vi "Com_SECS Equipment _Session Read.vi"(8 "error in":errorcluster, 10 "Timeout(100)":i32=100, 11 "Session In":refnum<k5>) -> (0 "error out":errorcluster, 2 "Read Data":string, 3 "Session Out":refnum<k5>)   [LabVIEW 2016]
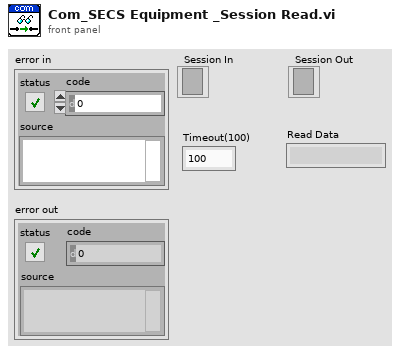
[diagram p1: front panel]
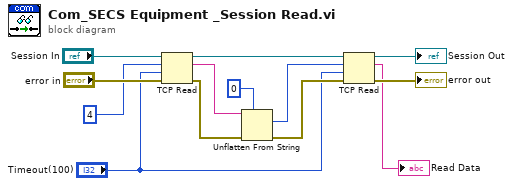
[diagram p0: block diagram]
diagram:
  n1 = TCP Read(connection ID="Session In", bytes to read=4, error in (no error)="error in", 9:"Timeout(100)") -> (connection ID out=w7:refnum<k5>, data out=w8:string, error out=w9:errorcluster)  [unwired: 1 out]
  n2 = Unflatten From String(type=0 ("bytes to read"), binary string=w8, error in (no error)=w9) -> (value=w6:i32, error out=w5:errorcluster)  [unwired: 1 in, 2 out]
  n3 = TCP Read(connection ID=w7, bytes to read=w6, error in (no error)=w5, 9:"Timeout(100)") -> (connection ID out=→"Session Out":refnum<k5>, data out=→"Read Data":string, error out=→"error out":errorcluster)  [unwired: 1 out]
